vi "Read Allow Undefinded Values.vi"(9 "Combobox in":refnum<class "Combobox.lvclass">) -> (3 "Combobox out":refnum<class "Combobox.lvclass">, 4 "Allow Undefinded Values":bool)   [LabVIEW 2014, in "Raspberry Pi Compatible Compiler for LabVIEW.lvlib" / "Combobox.lvclass"]
uses:
  Combobox.lvclass
  Combobox.lvclass/Combobox.ctl
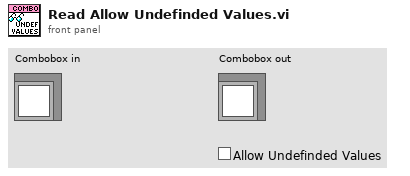
[diagram p1: front panel]
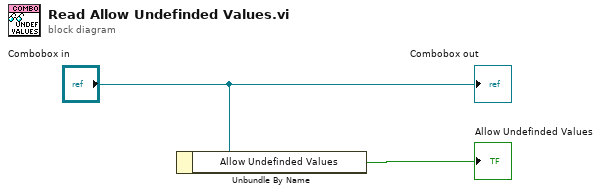
[diagram p0: block diagram]
diagram:
  n1 = Unbundle By Name("Combobox in") -> ("Allow Undefinded Values"=→"Allow Undefinded Values":bool)
  "Combobox out" <- "Combobox in"
